vi "Actor Core.vi"(8 "error in":errorcluster, 11 "Hardware Screen Interface in":refnum<class "Hardware Screen Interface.lvclass">) -> (0 "error out":errorcluster, 3 "Actor out":refnum<class "Actor.lvclass">)   [LabVIEW 2017, in "Hardware Screen Interface.lvlib" / "Hardware Screen Interface.lvclass"]
doc: "(<B>Filename</B>: Actor Framework.lvlib:Actor.lvclass:Actor Core.vi)\n\nReceives messages to the actor, reacts to them, and initiates any error handling that may shut the actor down.\n\nDescendant classes may override this VI to append parallel tasks for the actor to complete while it handles messages. Overrides use the Call Parent Method node."
uses:
  Hardware Screen Interface.lvclass
  Screen Interface/Screen Interface/Screen Interface.lvclass
  <vilib>/rvi/interface/nirviOpenFPGA/nirviOpenFPGA.xnode
  FPGA Bitfiles/WearableTetris_FPGATarget_OutputStream_Xjt08zbXoMY.lvbitx
  FPGA Code/Output Pulse Train.vi
  <vilib>/FPGAPlugInAG/myRIO-1900/niLvFpga_Open_myRIO-1900.vi
  <vilib>/rvi/interface/common/dynamic/niFpgaDynamicAddResources.vi
  <vilib>/ActorFramework/Actor/Actor.lvclass
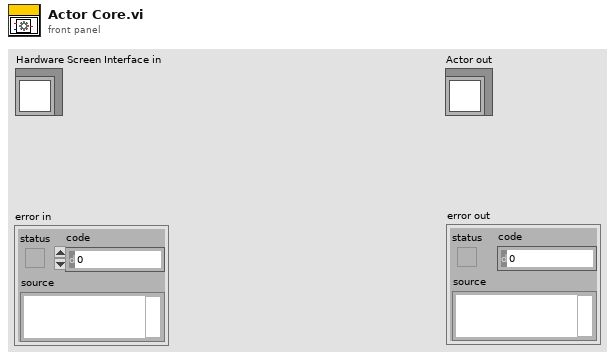
[diagram p1: front panel]
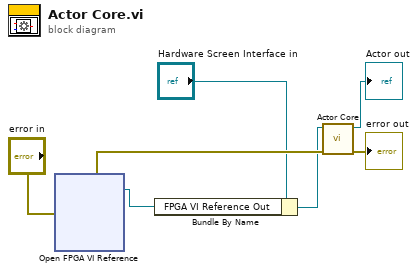
[diagram p0: block diagram]
diagram:
  n1 = xnode "Open FPGA VI Reference"("error in"="error in") -> ("FPGA VI Reference Out"=w5:refnum<k20>, "error out"=w3:errorcluster)  [unwired: 1 in]
  n2 = Bundle By Name(cluster="Hardware Screen Interface in", "FPGA VI Reference Out"=w5) -> (w1:refnum<class "Hardware Screen Interface.lvclass">)
  n3 = call-parent "Actor Core.vi"("error in"=w3, "Screen Interface in"=w1) -> ("error out"=→"error out":errorcluster, "Actor out"=→"Actor out":refnum<class "Actor.lvclass">)  [unwired: 8 in]
